vi "Simple Local Test.vi"() -> ()   [LabVIEW 2020]
uses:
  Stream-TCP/TCP Server/TCP Server.lvclass
  C:/dev/LabVIEW/lv-stream/stream/Endpoint/Endpoint.lvclass
  Stream-TCP/TCP Client/TCP Client.lvclass
  lv-stream/stream/Stream/Stream.lvclass
  lv-stream/stream/Endpoint/Endpoint.lvclass
panel:
  out "Client Error":errorcluster
  out "Server Error":errorcluster
  out "Message":string
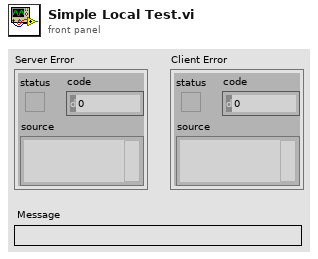
[diagram p1: front panel]
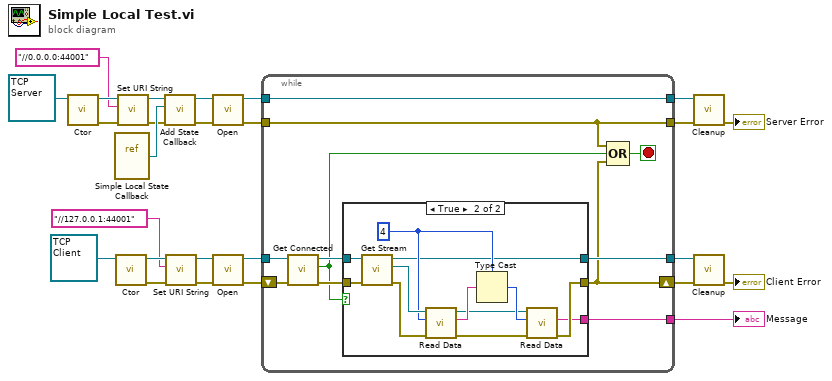
[diagram p0: block diagram]
diagram:
  n1 = call-dynamic "Ctor.vi"("TCP Server in"=refnum<class "TCP Server.lvclass"> refnum) -> ("error out"=w22:errorcluster, "TCP Server out"=w26:refnum<class "TCP Server.lvclass">)  [unwired: 9 in]
  n2 = vi-ref "Simple Local State Callback.vi"() -> (w23:refnum<vi>)
  n3 = call-dynamic "Ctor.vi"("TCP Client in"=refnum<class "TCP Client.lvclass"> refnum ("Stream-TCP.lvlib:TCP Client.lvclass")) -> ("error out"=w17:errorcluster, "TCP Client out"=w16:refnum<class "TCP Client.lvclass">)  [unwired: 9 in]
  n4 = call "Set URI String.vi"("error in (no error)"=w22, "URI String"="//0.0.0.0:44001", "Endpoint in"=w26) -> ("error out"=w21:errorcluster, "Endpoint out"=w24:refnum<class "TCP Server.lvclass">)  [unwired: 7 in]
  n5 = call-dynamic "Add State Callback.vi"("error in (no error)"=w21, "Callback"=w23, "Endpoint in"=w24) -> ("error out"=w18:errorcluster, "Endpoint out"=w19:refnum<class "TCP Server.lvclass">)  [unwired: 7 in]
  n6 = call "Set URI String.vi"("error in (no error)"=w17, "URI String"="//127.0.0.1:44001", "Endpoint in"=w16) -> ("error out"=w12:errorcluster, "Endpoint out"=w13:refnum<class "TCP Client.lvclass">)  [unwired: 7 in]
  n7 = call-dynamic "Open.vi"("error in (no error)"=w18, "TCP Server in"=w19) -> ("error out"=w8:errorcluster, "TCP Server out"=w9:refnum<class "TCP Server.lvclass">)  [unwired: 8 in]
  n8 = call-dynamic "Open.vi"("error in (no error)"=w12, "TCP Client in"=w13) -> ("error out"=w10:errorcluster, "TCP Client out"=w11:refnum<class "TCP Client.lvclass">)  [unwired: 8 in]
  n9 = while {
    tunnel: w11 -> [w37]
    tunnel: w9 -> [w31]
    shift-right: [w29] -> w5
    shift-left: w10 -> [w36]
    tunnel: [w33] -> w7
    tunnel: [w32] -> w6
    tunnel: [w31] -> w4
    tunnel: w8 -> [w28]
    tunnel: [w28] -> w3
    stop <- w27 stop-if-true
    n10 = call-dynamic "Get Connected.vi"("error in (no error)"=w36, "TCP Client in"=w37) -> ("error out"=w35:errorcluster, "Connected"=w30:bool, "TCP Client out"=w34:refnum<class "TCP Client.lvclass">)  [unwired: 7 in]
    n11 = case shown="True" w30 {
      tunnel: w35 -> [w39 w47]
      tunnel: w34 -> [w38 w48]
      tunnel: [_ w41] -> w33
      tunnel: [w39 w51] -> w29
      tunnel: [w38 w40] -> w32
      frame False {
      }
      frame True {
        w44 = 4 ("Count")
        n12 = call-dynamic "Get Stream.vi"("error in (no error)"=w47, "TCP Client in"=w48) -> ("error out"=w49:errorcluster, "Stream"=w46:refnum<class "Stream.lvclass">, "TCP Client out"=w40:refnum<class "TCP Client.lvclass">)  [unwired: 7 in]
        n13 = call-dynamic "Read Data.vi"("error in (no error)"=w49, "Count"=w44, "Stream in"=w46) -> ("error out"=w50:errorcluster, "Data"=w45:string, "Stream out"=w42:refnum<class "Stream.lvclass">)  [unwired: 6 in]
        n14 = Type Cast(type=w44, x=w45) -> (*(type *) &x=w43:i32)
        n15 = call-dynamic "Read Data.vi"("error in (no error)"=w50, "Count"=w43, "Stream in"=w42) -> ("error out"=w51:errorcluster, "Data"=w41:string)  [unwired: 6 in, 1 out]
      }
    }
    n16 = Compound Arithmetic op=OR(w28, w30, w29) -> (w27:bool)
  }
  "Message" <- w7
  n17 = call-dynamic "Cleanup.vi"("error in (no error)"=w3, "TCP Server in"=w4) -> ("error out"=→"Server Error":errorcluster)  [unwired: 9 in]
  n18 = call-dynamic "Cleanup.vi"("error in (no error)"=w5, "TCP Client in"=w6) -> ("error out"=→"Client Error":errorcluster)  [unwired: 9 in]
